vi "GetElement(Single).vi"(7 "Qualified Name":string, 8 "error in (no error)":errorcluster, 10 "Key":string, 11 "ConfigManager.Text in":refnum<class "ConfigManager.Text.lvclass">) -> (0 "error out":errorcluster, 1 "found":bool, 2 "Value":string, 3 "ConfigManager.Text out":refnum<class "ConfigManager.Text.lvclass">)   [LabVIEW 2013, in "CfgManager.Text.lvlib" / "ConfigManager.Text.lvclass"]
uses:
  ConfigManager.Text.lvclass
  ConfigManager.Text.lvclass/ConfigManager.Text.ctl
  Response - cluster.ctl
  Query -- cluster.ctl
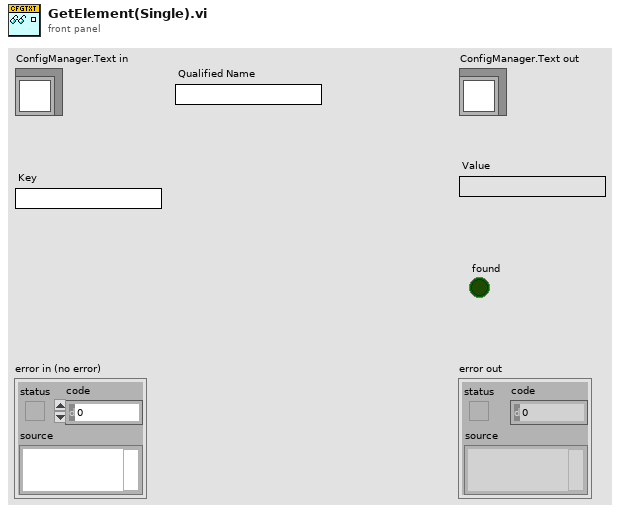
[diagram p1: front panel]
types:
  T1 = typedef "CfgManager.Text.lvlib/ConfigManager.Text.lvclass/Query -- cluster.ctl" = cluster{"Qualified Name":string[], "Keys":string[]}
  T2 = typedef "CfgManager.Text.lvlib/ConfigManager.Text.lvclass/Response - cluster.ctl" = cluster{"Keys":string[], "Values":string[], "Found":bool[]}
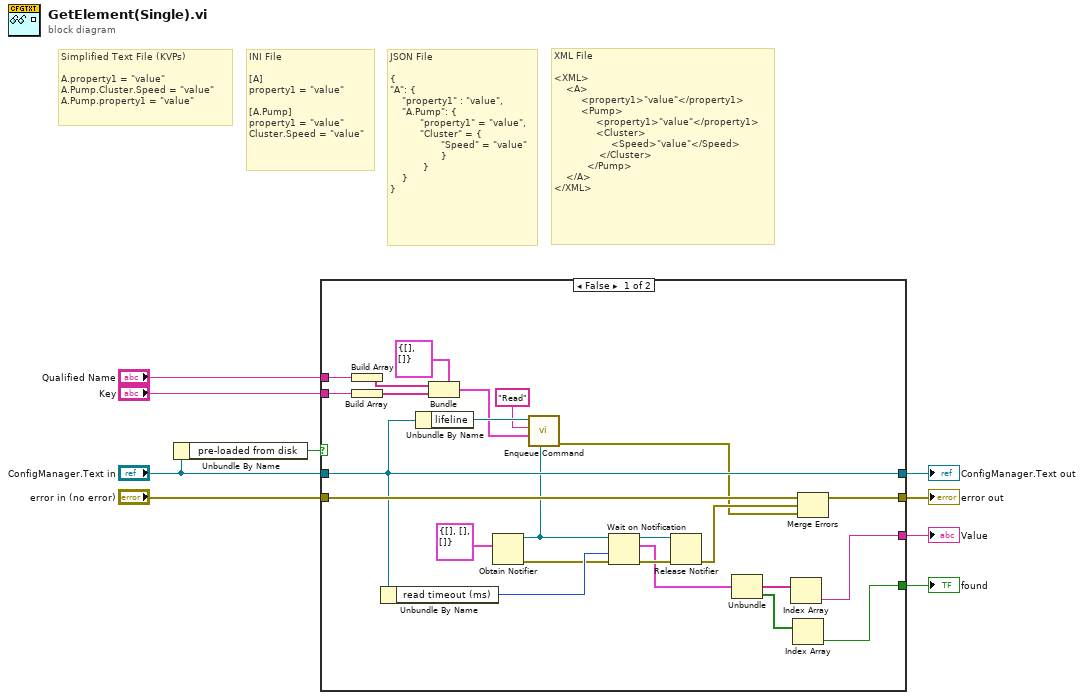
[diagram p0: block diagram]
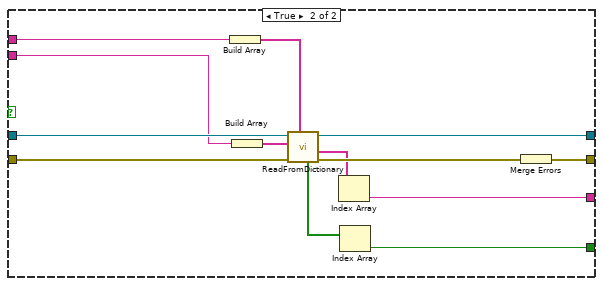
[diagram p2: hidden frame]
diagram:
  # "XML File\n\n<XML>\n    <A>\n         <property1>\"value\"</property1>\n         <Pump> \n              <property1>\"value\"</property1>\n              <Cluster>\n                   <Speed>\"value\"</Speed>\n               </Cluster>  \n           </Pump>\n    </A>\n</XML>"
  # "JSON File\n\n{\n\"A\": {\n    \"property1\" : \"value\",\n    \"A.Pump\": {\n          \"property1\" = \"value\",\n          \"Cluster\" = {\n                 \"Speed\" = \"value\"\n                 }\n           }\n    }\n}"
  # "INI File\n\n[A]\nproperty1 = \"value\"\n\n[A.Pump]\nproperty1 = \"value\"\nCluster.Speed = \"value\""
  # "Simplified Text File (KVPs)\n\nA.property1 = \"value\"\nA.Pump.Cluster.Speed = \"value\"\nA.Pump.property1 = \"value\""
  n1 = Unbundle By Name("ConfigManager.Text in") -> ("pre-loaded from disk"=w1:bool)
  n2 = case shown="False" w1 {
    tunnel: [w24 w46] -> w9
    tunnel: [w18 w36] -> w8
    tunnel: [w22 w40] -> w7
    tunnel: [w14 w42] -> w6
    tunnel: "Qualified Name" -> [w11 w35]
    tunnel: "error in (no error)" -> [w26 w45]
    tunnel: "Key" -> [w32 w41]
    tunnel: "ConfigManager.Text in" -> [w14 w43]
    frame False {
      n3 = Build Array(w11) -> (w10:string[])
      n4 = Build Array(w32) -> (w21:string[])
      n5 = Unbundle By Name(w14) -> ("read timeout (ms)"=w28:i32)
      n6 = Unbundle By Name(w14) -> ("lifeline"=w17:refnum<queue>)
      n7 = Bundle(cluster=T1 {"Qualified Name"=[], "Keys"=[]} ("Query"), "Qualified Name"=w10, "Keys"=w21) -> (w15:T1)
      n8 = Obtain Notifier(notification data type=T2 {"Keys"=[], "Values"=[], "Found"=[]} ("response")) -> (notifier out=w13:refnum<notifier>, error out=w27:errorcluster)  [unwired: 3 in, 1 out]
      n9 = call "Enqueue Command.vi"("query notifier"=w13, "args"=w15, "command"="Read", "Queue in"=w17) -> ("error out"=w12:errorcluster)  [unwired: 5 in, 2 out]
      n10 = Wait on Notification(notifier=w13, timeout in ms (-1)=w28, error in (no error)=w27) -> (notifier out=w30:refnum<notifier>, notification=w23:T2, error out=w29:errorcluster)  [unwired: 1 in, 1 out]
      n11 = Release Notifier(notifier=w30, error in (no error)=w29) -> (error out=w25:errorcluster)  [unwired: 1 in, 2 out]
      n12 = Unbundle(w23) -> ("Values"=w20:string[], "Found"=w19:bool[])  [unwired: 1 out]
      n13 = Index Array(array=w20) -> (element=w22:string)  [unwired: 1 in]
      n14 = Index Array(array=w19) -> (element=w18:bool)  [unwired: 1 in]
      n15 = Merge Errors(w26, w25, w12) -> (w24:errorcluster)
    }
    frame True {
      n16 = Build Array(w35) -> (w34:string[])
      n17 = Build Array(w41) -> (w38:string[])
      n18 = call "ReadFromDictionary.vi"("Qualified Name"=w34, "error in (no error)"=w45, "Keys"=w38, "ConfigManager.Text in"=w43) -> ("error out"=w44:errorcluster, "Values"=w39:string[], "ConfigManager.Text out"=w42:refnum<class "ConfigManager.Text.lvclass">, "Found"=w37:bool[])  [unwired: 3 in, 1 out]
      n19 = Index Array(array=w39) -> (element=w40:string)  [unwired: 1 in]
      n20 = Index Array(array=w37) -> (element=w36:bool)  [unwired: 1 in]
      n21 = Merge Errors(w44) -> (w46:errorcluster)
    }
  }
  "error out" <- w9
  "ConfigManager.Text out" <- w6
  "Value" <- w7
  "found" <- w8
